vi "TRANSPOSED_VERTREAD_CSV_import_control_lasers_and_SMs_and_ICC4C_Cam_Trigger_Older.vi"() -> ()   [LabVIEW 2021]
uses:
  <vilib>/DAQmx/write.llb/DAQmx Write (Analog 1D DBL NChan 1Samp).vi
  <vilib>/DAQmx/create/channels.llb/DAQmx Create Channel (AO-Voltage-Basic).vi
  <vilib>/Utility/file.llb/Read Delimited Spreadsheet (DBL).vi
  <vilib>/DAQmx/miscellaneous.llb/DAQmx Fill In Error Info.vi
panel:
  out "MINIMUM DELAY":dbl
  out "Raw  Inner Loop Iternation":dbl
  out "CamTriggerStatus":dbl
  out "Trigger_Phase_Iterations":i32
  out "Cam_Trigger_Lo":dbl
  out "Cam_Trigger_Hi":dbl
  out "Sequence Length":i32
  in  "Delay (> Minimum)":i32
  in  "ICC4C 3 (0-10V)":dbl
  in  "ICC4C 2 (0-10V)":dbl
  in  "ICC4C 1 (0-10V)":dbl
  in  "ICC4C 0 (0-10V)":dbl
  in  "Y2 (-10-10V)":dbl
  in  "X2 (-10-10V)":dbl
  in  "Continue Cycle?":bool
  out "Full Cycles":i32
  out "Mirror_Phase_Iterations":i32
  out "Y1 (-10-10V)":dbl format="%_6g"
  out "X1 (-10-10V)":dbl format="%_6g"
  in  "Blanking (0-10v)":dbl=10.0
  in  "561 (0-10v)":dbl
  in  "514 (0-10v)":dbl
  in  "488 (0-10v)":dbl
  in  "445 (0-10v)":dbl
  # "NOTE: CURRENTLY DROPS FIRST IMAGE DUE TO ANDOR TRIGGERING ON SECOND AQUISITION ONLY"
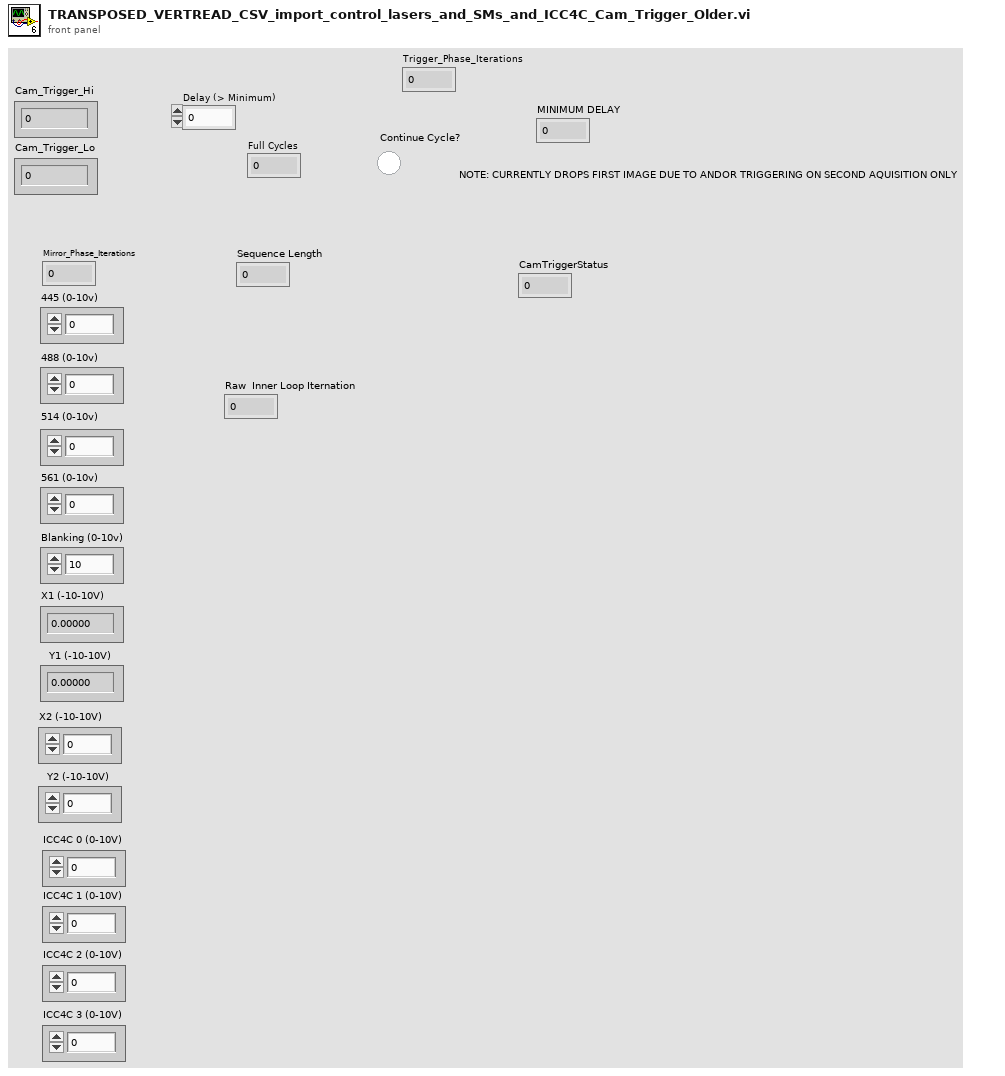
[diagram p1: front panel]
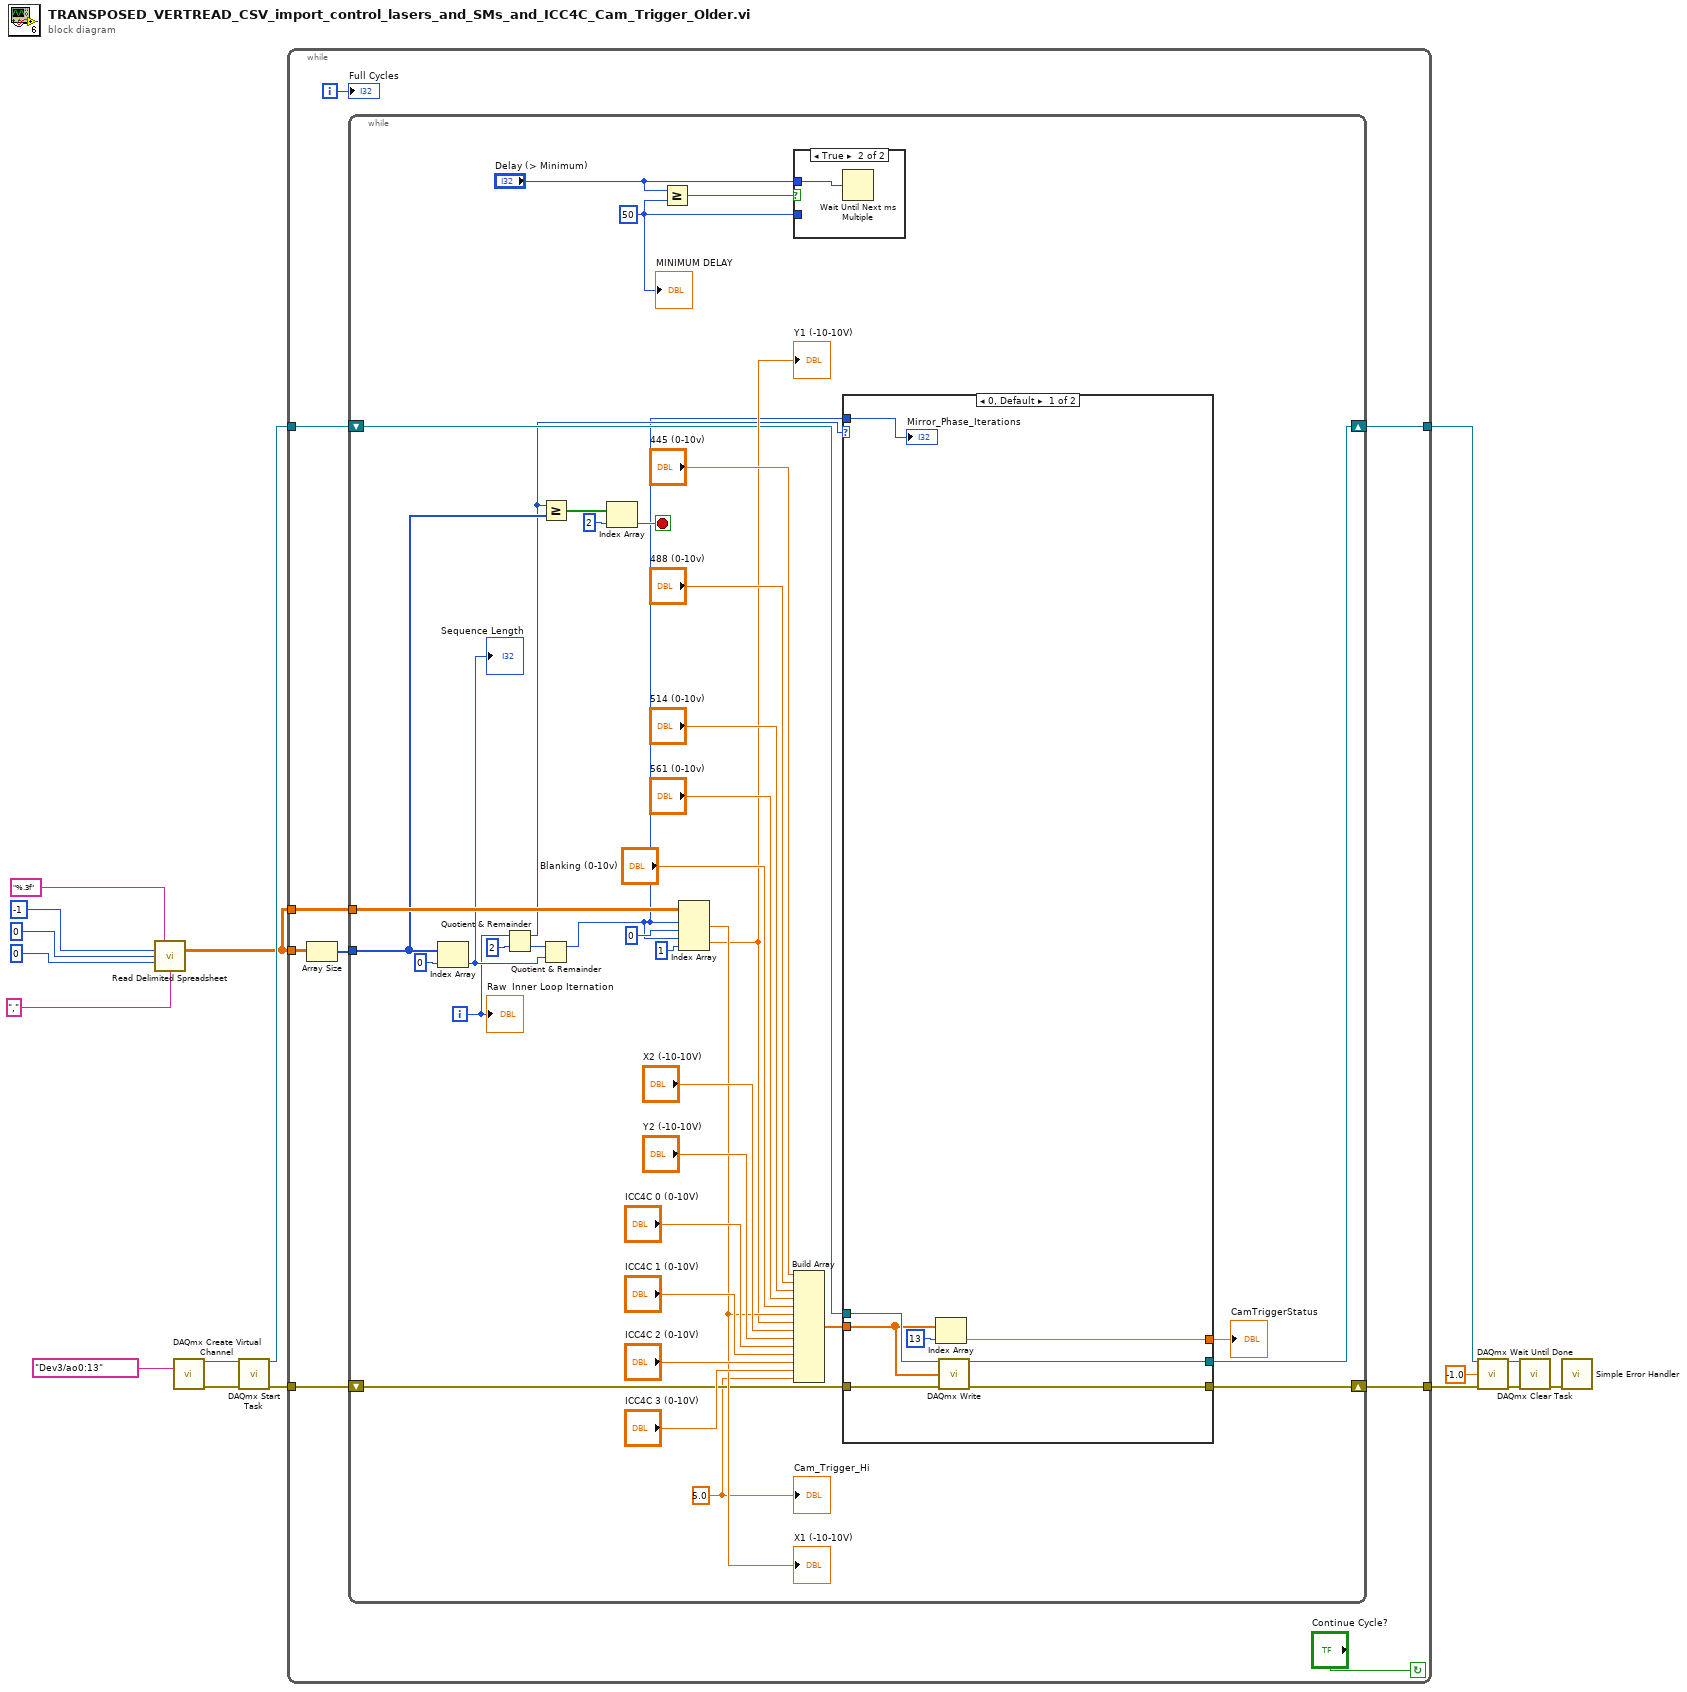
[diagram p0: block diagram]
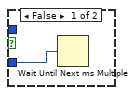
[diagram p2: hidden frame]
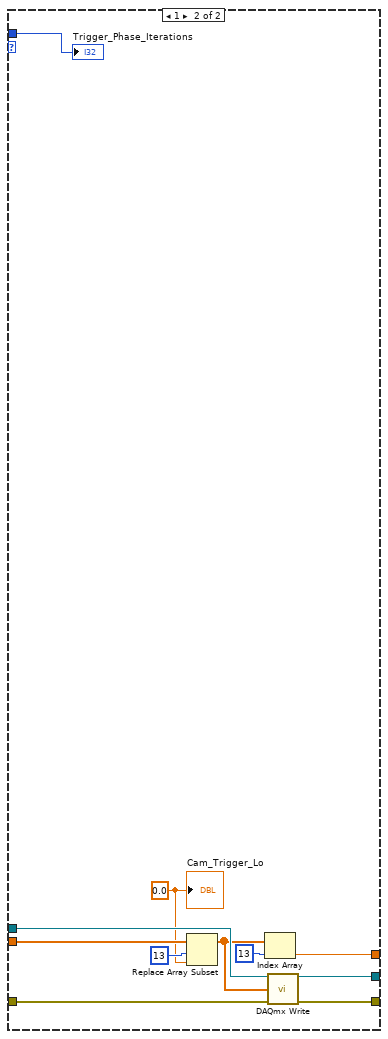
[diagram p3: hidden frame]
diagram:
  n1 = call-poly <vilib>:"Read Delimited Spreadsheet.vi"("format (%.3f)"="%.3f", "number of rows (all:-1)"=-1, "start of read offset (chars.:0)"=0, "max characters/row  (no limit:0)"=0, "delimiter (\\t)"=",") -> ("all rows"=w6:dbl[][])  [unwired: 5 in, 5 out]
  n2 = call-poly <vilib>:"DAQmx Create Virtual Channel.vi"("physical channels"=tag "Dev3/ao0:13") -> ("task out"=w10:refnum<k21>, "error out"=w9:errorcluster)  [unwired: 13 in]
  n3 = call <vilib>:"DAQmx Start Task.vi"("task/channels in"=w10, "error in"=w9) -> ("task out"=w8:refnum<k21>, "error out"=w7:errorcluster)  [unwired: 12 in]
  n4 = while {
    tunnel: [w23] -> w13
    tunnel: [w22] -> w12
    tunnel: w8 -> [w25]
    tunnel: w7 -> [w24]
    tunnel: w6 -> [w20]
    tunnel: w6 -> [w19]
    i -> [w26]
    stop <- "Continue Cycle?" continue-if-true
    n5 = Array Size(array=w20) -> (size(s)=w21:i32[])
    n6 = while {
      shift-right: [w41] -> w23
      shift-left: w25 -> [w39]
      shift-right: [w42] -> w22
      shift-left: w24 -> [w38]
      tunnel: w21 -> [w47]
      tunnel: w19 -> [w49]
      i -> [w30]
      stop <- w50 stop-if-true
      w27 = 50
      w31 = 5.0
      n7 = Index Array(array=w47, index=0) -> (element=w45:i32)
      "Sequence Length" <- w45
      n8 = Quotient & Remainder(x=w30, y=2) -> (x-y*floor(x/y)=w36:i32, floor(x/y)=w35:i32)
      n9 = Greater Or Equal?(x=w36, y=w47) -> (x >= y?=w51:bool[])
      n10 = Quotient & Remainder(x=w35, y=w45) -> (x-y*floor(x/y)=w32:i32)  [unwired: 1 out]
      n11 = Index Array(array=w51, index=2) -> (element=w50:bool)
      n12 = Greater Or Equal?(x="Delay (> Minimum)", y=w27) -> (x >= y?=w28:bool)
      n13 = Index Array(array=w49, index (row) #1=w32, index (col) #1=0, index (row) #2=w32, index (col) #2=1) -> (element #1=w52:dbl, element #2=w48:dbl)
      "X1 (-10-10V)" <- w52
      "Y1 (-10-10V)" <- w48
      n14 = case shown="True" w28 {
        tunnel: "Delay (> Minimum)" -> [_ w65]
        tunnel: w27 -> [w64 _]
        frame False {
          n15 = Wait Until Next ms Multiple(millisecond multiple=w64) -> ()  [unwired: 1 out]
        }
        frame True {
          n16 = Wait Until Next ms Multiple(millisecond multiple=w65) -> ()  [unwired: 1 out]
        }
      }
      n17 = Build Array("445 (0-10v)", "488 (0-10v)", "514 (0-10v)", "561 (0-10v)", "Blanking (0-10v)", w52, w48, "X2 (-10-10V)", "Y2 (-10-10V)", "ICC4C 0 (0-10V)", "ICC4C 1 (0-10V)", "ICC4C 2 (0-10V)", "ICC4C 3 (0-10V)", w31) -> (w43:dbl[])
      n18 = case shown="0, Default" w36 {
        tunnel: w39 -> [w73 w84]
        tunnel: [w70 w83] -> w41
        tunnel: w38 -> [w72 w82]
        tunnel: [w71 w78] -> w42
        tunnel: w43 -> [w69 w81]
        tunnel: w32 -> [w66 w79]
        tunnel: [w67 w75] -> w37
        frame 0, Default {
          n19 = Index Array(array=w69, index=13) -> (element=w67:dbl)
          n20 = call-poly <vilib>:"DAQmx Write.vi"("task/channels in"=w73, "data"=w69, "error in"=w72) -> ("task out"=w70:refnum<k21>, "error out"=w71:errorcluster)  [unwired: 10 in, 1 out]
          "Mirror_Phase_Iterations" <- w66
        }
        frame 1 {
          w74 = 0.0
          n21 = Replace Array Subset(array=w81, new element=w74, index=13) -> (w76:dbl[])
          n22 = Index Array(array=w76, index=13) -> (element=w75:dbl)
          n23 = call-poly <vilib>:"DAQmx Write.vi"("task/channels in"=w84, "data"=w76, "error in"=w82) -> ("task out"=w83:refnum<k21>, "error out"=w78:errorcluster)  [unwired: 10 in, 1 out]
          "Cam_Trigger_Lo" <- w74
          "Trigger_Phase_Iterations" <- w79
        }
      }
      "CamTriggerStatus" <- w37
      "Cam_Trigger_Hi" <- w31
      "Raw  Inner Loop Iternation" <- w30
      "MINIMUM DELAY" <- w27
    }
    "Full Cycles" <- w26
  }
  n24 = call <vilib>:"DAQmx Wait Until Done.vi"("task/channels in"=w13, "timeout (sec)"=-1.0, "error in"=w12) -> ("task out"=w16:refnum<k21>, "error out"=w15:errorcluster)  [unwired: 11 in]
  n25 = call <vilib>:"DAQmx Clear Task.vi"("task in"=w16, "error in"=w15) -> ("error out"=w17:errorcluster)  [unwired: 13 in]
  n26 = call <vilib>:"Simple Error Handler.vi"("error in (no error)"=w17) -> ()  [unwired: 4 in, 5 out]
